vi "Windows UI.vi"() -> ()   [LabVIEW 2014]
doc: "This is the primary Host VI."
panel:
  in  "IP Address NOTE: Update with your eval device IP address and select Edit>>Make Current Values Default before running":string="10.0.0.2"
  out "Display Battery State":bool
  out "Current Temperature":dbl(knob) scale=20.0..40.0
  out "Battery State":enum16{"Charged", "Running", "Low Batt"}(ring)
  out "Display RPM":bool
  out "Display Temperature":bool
  out "Display Voltage":bool
  out "Temperature Warning":bool
  out "Current RPM":dbl(knob) scale=0.0..1000.0
  in  "Stop Button":bool
  out "Error Out":errorcluster
  out "Current Voltage":dbl(knob) scale=0.0..4.0
  out "Variable History":cluster{dbl, dbl, dbl}(graph)
  # "LCD Controls"
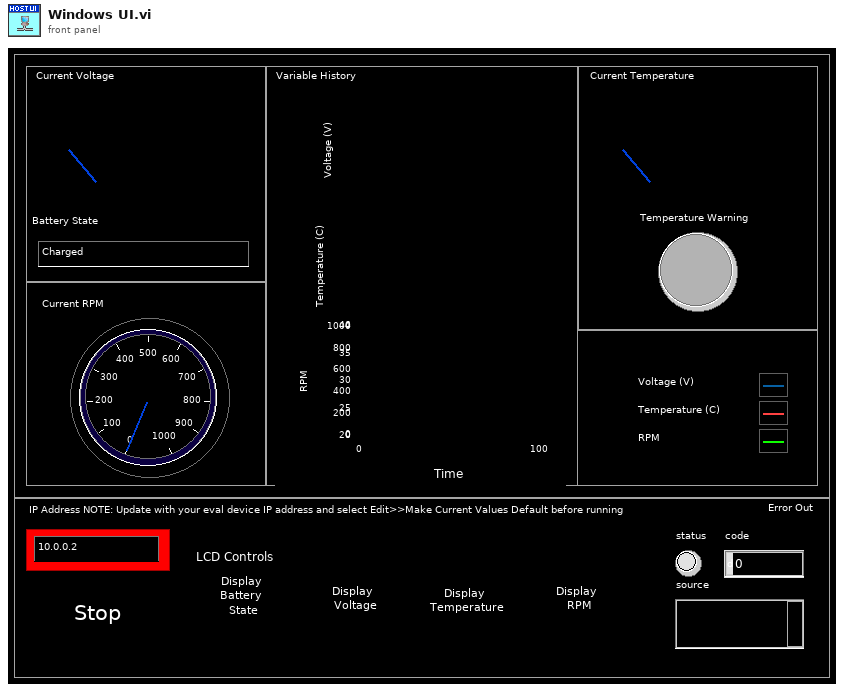
[diagram p1: front panel]
types:
  T1 = cluster{"Temperature Ref":refnum<k21>, "Temperature Warning Ref":refnum<k21>, "Voltage Ref":refnum<k21>, "Battery State Ref":refnum<k21>, "RPM Ref":refnum<k21>, "Display State Ref":refnum<k21>}
  T2 = typedef "Display State.ctl" = enum16{"Battery State", "RPM", "Temp", "Voltage"}
  T3 = cluster{"Temperature":fxp<+/-,32,13>, "Temperature Warning":bool, "Voltage":fxp<+/-,24,5>, "Battery State":enum16{"Charged", "Running", "Low Batt"}, "RPM":fxp<+,32,16>, "Display State":T2}
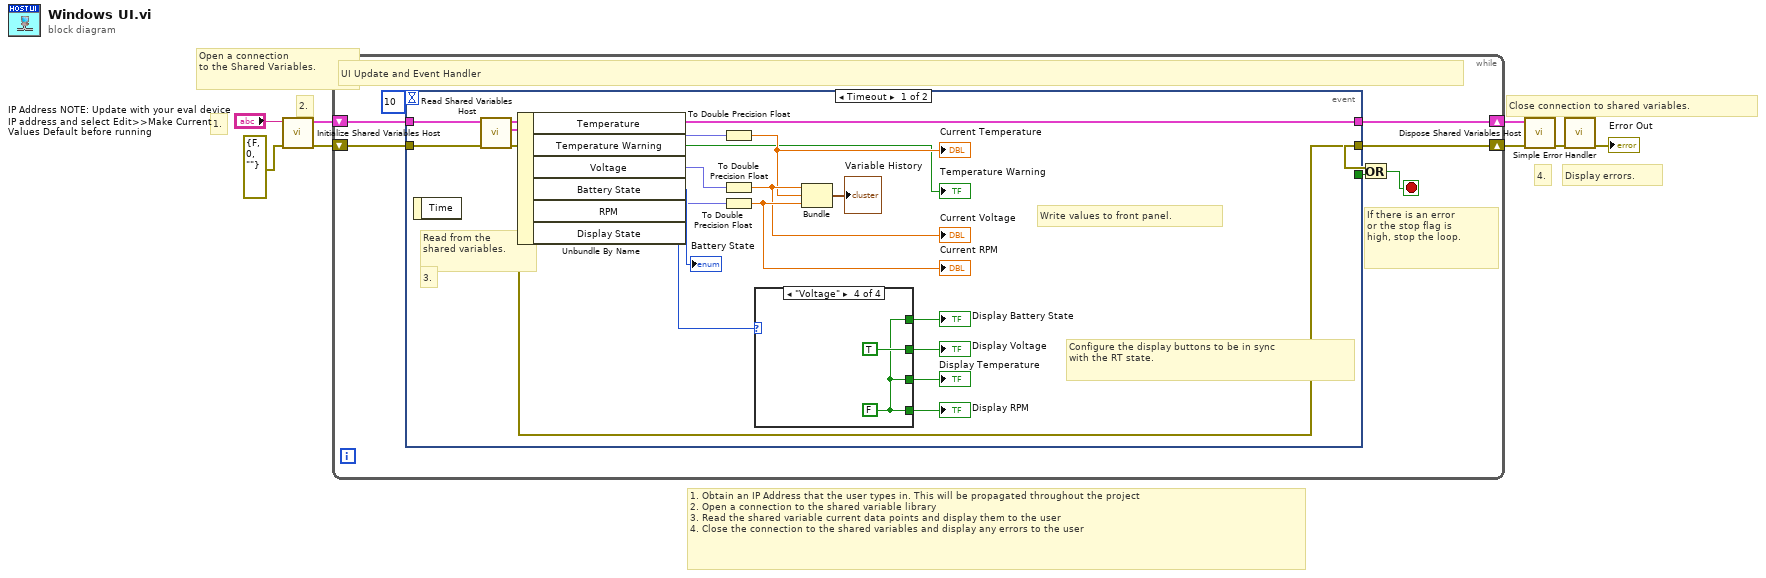
[diagram p0: block diagram]
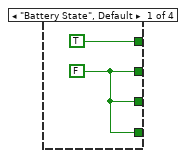
[diagram p2: hidden frame]
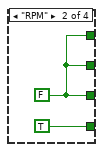
[diagram p3: hidden frame]
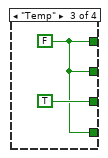
[diagram p4: hidden frame]
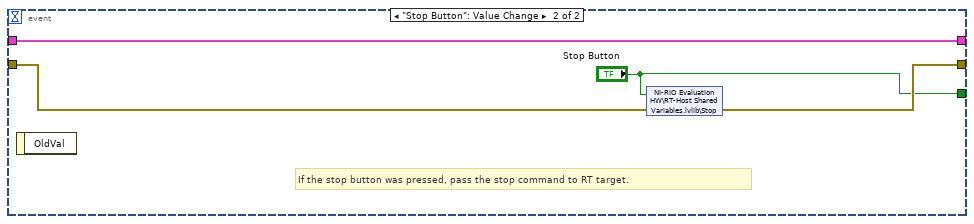
[diagram p5: hidden frame]
diagram:
  # "1. Obtain an IP Address that the user types in. This will be propagated throughout the project\n2. Open a connection to the shared variable library\n3. Read the shared variable current data points and display them to the user\n4. Close the connection to the shared variables and display any errors to the user"
  # "4."
  # "2."
  # "1."
  # "Close connection to shared variables."
  # "Display errors."
  # "Open a connection\nto the Shared Variables."
  n1 = call "Initialize Shared Variables Host.vi"("error in (no error)"=errorcluster {"status"=FALSE, "code"=0, "source"=""} ("error out"), "IP Address (No Slashes)"="IP Address NOTE: Update with your eval device IP address and select Edit>>Make Current Values Default before running") -> ("error out"=w7:errorcluster, "Shared Variable References"=w8:T1)  [unwired: 8 in]
  n2 = while {
    shift-right: [w10] -> w5
    shift-left: w7 -> [w15]
    shift-right: [w12] -> w6
    shift-left: w8 -> [w13]
    stop <- w11 stop-if-true
    # "UI Update and Event Handler"
    # "If there is an error\nor the stop flag is\nhigh, stop the loop."
    n3 = event shown="[0] Timeout" {
      selector: _ -> [_ _]
      dyn-events: _ -> [_ _]
      timeout: 10 -> [_ _]
      tunnel: [w21 w44] -> w10
      tunnel: w15 -> [w23 w45]
      tunnel: w13 -> [w30 w46]
      tunnel: [w16 w46] -> w12
      tunnel: [_ "Stop Button"] -> w9
      event Timeout {
        # "3."
        # "Write values to front panel."
        # "Read from the\nshared variables."
        # "Configure the display buttons to be in sync\nwith the RT state."
        n4 = event-data() -> ()  [unwired: 1 in, 1 out]
        n5 = call "Read Shared Variables Host.vi"("error in (no error)"=w23, "Shared Variable References"=w30) -> ("error out"=w21:errorcluster, "Current Values"=w22:T3, "Shared Variable References Out"=w16:T1)  [unwired: 7 in]
        n6 = Unbundle By Name(w22) -> ("Temperature"=w27:fxp<+/-,32,13>, "Temperature Warning"=→"Temperature Warning":bool, "Voltage"=w29:fxp<+/-,24,5>, "Battery State"=→"Battery State":enum16{"Charged", "Running", "Low Batt"}, "RPM"=w25:fxp<+,32,16>, "Display State"=w24:T2)
        n7 = To Double Precision Float(number=w27) -> (double precision float=w31:dbl)
        "Current Temperature" <- w31
        n8 = To Double Precision Float(number=w29) -> (double precision float=w32:dbl)
        "Current Voltage" <- w32
        n9 = To Double Precision Float(number=w25) -> (double precision float=w33:dbl)
        "Current RPM" <- w33
        n10 = case shown="\"Voltage\"" w24 {
          tunnel: [TRUE ("Display Battery State") w37 w39 w41] -> w20
          tunnel: [w35 w37 w39 TRUE ("Display Battery State")] -> w19
          tunnel: [w35 w37 TRUE ("Display Battery State") w41] -> w18
          tunnel: [w35 TRUE ("Display Battery State") w39 w41] -> w17
          frame "Battery State", Default {
            w35 = FALSE
          }
          frame "RPM" {
            w37 = FALSE
          }
          frame "Temp" {
            w39 = FALSE
          }
          frame "Voltage" {
            w41 = FALSE
          }
        }
        "Display Battery State" <- w20
        "Display Voltage" <- w19
        "Display Temperature" <- w18
        "Display RPM" <- w17
        n11 = Bundle(w32, w31, w33) -> (→"Variable History":cluster{dbl, dbl, dbl})  [unwired: 1 in]
      }
      event "Stop Button": Value Change {
        # "If the stop button was pressed, pass the stop command to RT target."
        n12 = event-data() -> ()  [unwired: 1 in, 1 out]
        n13 = shared-variable "NI-RIO Evaluation HW\\RT-Host Shared Variables.lvlib\\Stop"("Stop Button", error in=w45) -> (error out=w44:errorcluster)
      }
    }
    n14 = Or(x=w10, y=w9) -> (x .or. y?=w11:bool)
  }
  n15 = call "Dispose Shared Variables Host.vi"("error in (no error)"=w5, "Shared Variable References"=w6) -> ("error out"=w2:errorcluster)  [unwired: 9 in]
  n16 = call <vilib>:"Simple Error Handler.vi"("error in (no error)"=w2) -> ("error out"=→"Error Out":errorcluster)  [unwired: 4 in, 4 out]
